vi "SaveDeviceHeader.vi"(0 "File Refnum in":refnum<file>, 1 "Comments":string, 5 "Filename":string, 7 "Run Number":i32, 9 "Array Titles":string, 11 "error in (no error)":errorcluster, 12 "Temperature":dbl, 13 "Humidity":dbl, 14 "Strip Segment":string) -> (4 "File Refnum out":refnum<file>, 6 "Header string":string, 10 "error out":errorcluster)   [LabVIEW 2013]
uses:
  globals/QC_RunInformation.vi
  globals/QC_MeasurementSetup.vi
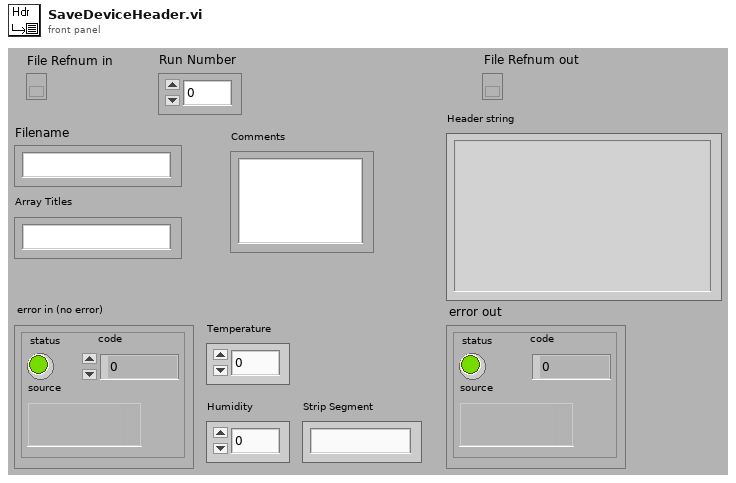
[diagram p1: front panel]
types:
  T1 = cluster{"Sensor Serial No.:":string, "Wafer:":string, "Batch:":string, "Manufacturer:":string, "Device Category:":string, "Database Serial No.:":string, "Date Initiated:":string, "Time Initiated:":string, "Test":string, "Probeplan used:":string, "End of Run comment:":string, "User:":string, "Vbias SMU":string, "LCR":string, "Test SMU":string, "Test DMM":string}
  T2 = cluster{"Institute":string, "Manufacturers":string[], "Devices":string[], "Serialnumbers Lookup DB":string, "Data directory":string, "Backup & screenshot directory":string, "List of known users":string[], "Measurement switch not used":bool, "Measurement Switch":string, "DUT Switch":string, "Rseries IV [MOhm]":string, "Rshunt IV [MOhm]":string, "Rseries CV [MOhm]":string, "DC blocking Cap [µF]":string, "Rseries LCR [MOhm]":string, "Rseries stability [MOhm]":string, "Rshunt stability [MOhm]":string, "Rseries striptest bias [MOhm]":string, "Rseries strip pinhole [MOhm]":string}
  T3 = cluster{"Supply":refnum<class "SupplyControl.lvclass">, "LCR":refnum<class "LCRControl.lvclass">, "Arduino":refnum<class "ArduinoControl.lvclass">, "Measurement switch":refnum<class "Switching.lvclass">, "Initial Voltage [V]":dbl, "Final Voltage [V]":dbl, "Step Size [V]":dbl, "Step Interval [s]":i32, "Number Of Steps":u32, "AC frequency [Hz]":i32, "RC Configuration":u16, "AC amplitude [V]":dbl, "Ramp down steps [V]":dbl, "Ramp down Interval [s]":i32, "Set Current Limit?":bool, "Current Limit [µA]":dbl, "Temperature Readout":enum16{"Read Arduino", "Enter manually"}, "Supply Name":string, "LCR Name":string, "V_depletion Limit [V]":dbl, "Measurement switch used?":bool}
  T4 = cluster{"Bias Supply":refnum<class "SupplyControl.lvclass">, "SMU":refnum<class "SupplyControl.lvclass">, "LCR":refnum<class "LCRControl.lvclass">, "ProbeStation":refnum<class "ProbeStationControl.lvclass">, "Arduino":refnum<class "ArduinoControl.lvclass">, "Measurement switch":refnum<class "Switching.lvclass">, "Probe Card Channels":i32, "Bias Voltage [V]":dbl, "First strip":i32, "Last strip":i32, "Base Voltage [V]":dbl, "Base Ramp Step [V]":dbl, "Base Ramp Interval [ms]":u32, "High Voltage [V]":dbl, "High Ramp Step [V]":dbl, "High Ramp Interval [ms]":u32, "AC frequency [Hz]":i32, "AC amplitude [V]":dbl, "RC Configuration":u16, "Single Needle":bool, "Temperature Readout":enum16{"Read Arduino", "Enter manually"}, "Fraction of good strips [%]":dbl, "Measurement switch used?":bool, "Matrix X Channels":cluster{"Mux1 C1":i32, "Mux1 C2":i32, "Mux2 C1":i32, "Mux2 C2":i32}, "Pinholes Y/N":bool, "Capacitance Y/N":bool, "Resistance Y/N":bool, "Bias Supply Name":string, "SMU Name":string, "LCR Name":string}
  T5 = cluster{"Supply":refnum<class "SupplyControl.lvclass">, "LCR":refnum<class "LCRControl.lvclass">, "Arduino":refnum<class "ArduinoControl.lvclass">, "Measurement switch":refnum<class "Switching.lvclass">, "Initial Voltage [V]":dbl, "Final Voltage [V]":dbl, "Step Size [V]":dbl, "Step Interval [s]":i32, "Number Of Steps":u32, "AC frequency [Hz]":i32, "RC Configuration":u16, "AC amplitude [V]":dbl, "Ramp down steps [V]":dbl, "Ramp down Interval [s]":i32, "Set Current Limit?":bool, "Current Limit [µA]":dbl, "Temperature Readout":enum16{"Read Arduino", "Enter manually"}, "Supply Name":string, "LCR Name":string, "C_is Limit [pF/cm]":dbl, "Measurement switch used?":bool}
  T6 = cluster{"Bias Supply":refnum<class "SupplyControl.lvclass">, "SMU":refnum<class "SupplyControl.lvclass">, "Arduino":refnum<class "ArduinoControl.lvclass">, "Initial Voltage [V]":dbl, "Final Voltage [V]":dbl, "Step Size [V]":dbl, "Step Interval [s]":i32, "Number Of Steps":u32, "Ramp down steps [V]":dbl, "Ramp down Interval [s]":i32, "Bias Voltage [V]":dbl, "Set Current Limit?":bool, "Current Limit [µA]":dbl, "Temperature Readout":enum16{"Read Arduino", "Enter manually"}, "Bias Supply Name":string, "SMU Name":string}
  T7 = cluster{"Supply":refnum<class "SupplyControl.lvclass">, "DMM":refnum<class "MultimeterControl.lvclass">, "DUT switch":refnum<class "Switching.lvclass">, "Arduino":refnum<class "ArduinoControl.lvclass">, "Measurement switch":refnum<class "Switching.lvclass">, "Voltage [V]":dbl, "Measurement Interval [s]":i32, "Test Duration":u32, "Ramp up steps [V]":dbl, "Ramp up Interval [s]":u32, "Ramp down steps [V]":dbl, "Ramp down Interval [s]":i32, "Set Current Limit?":bool, "Current Limit [µA]":dbl, "Temperature Readout":enum16{"Read Arduino", "Enter manually"}, "Supply Name":string, "DMM Name":string, "Maximum current fluctuation [%]":dbl, "Measurement switch used?":bool, "DUT switch used?":bool}
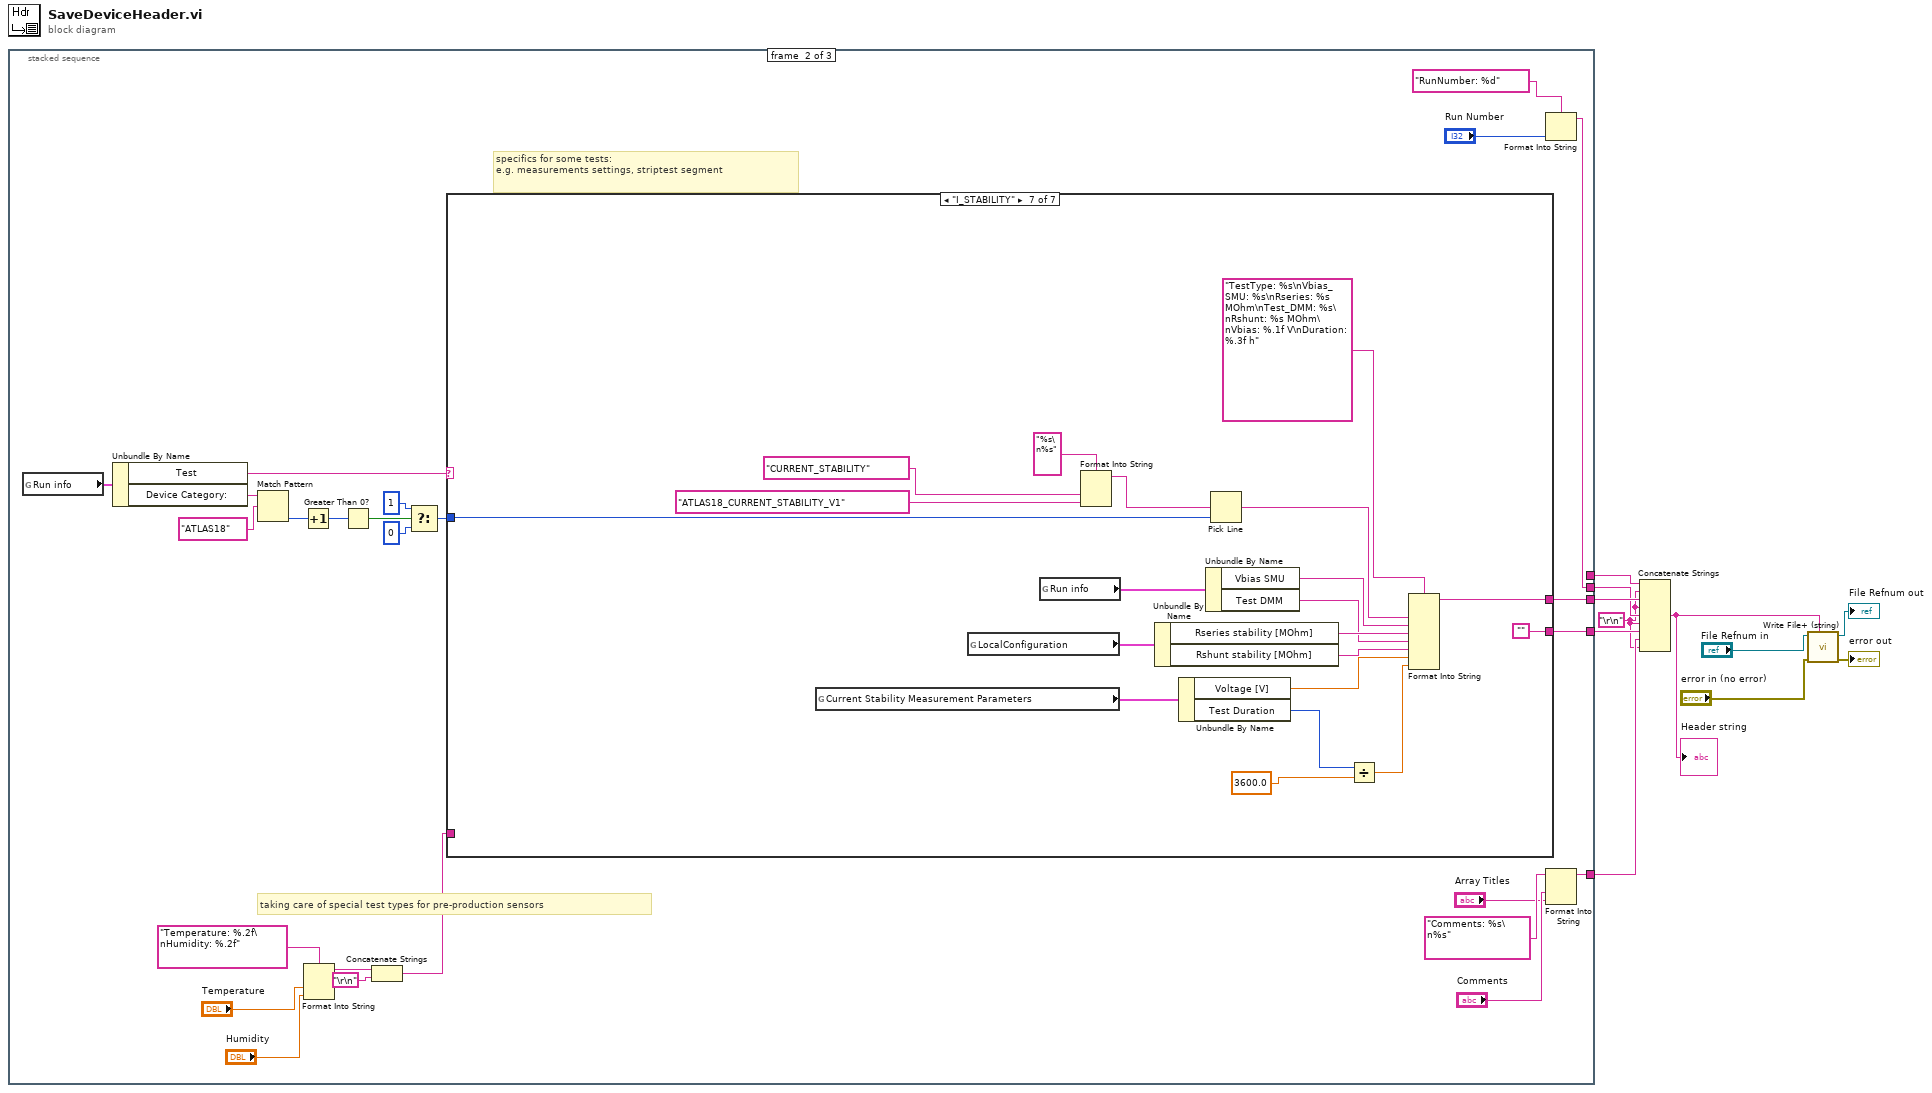
[diagram p0: block diagram]
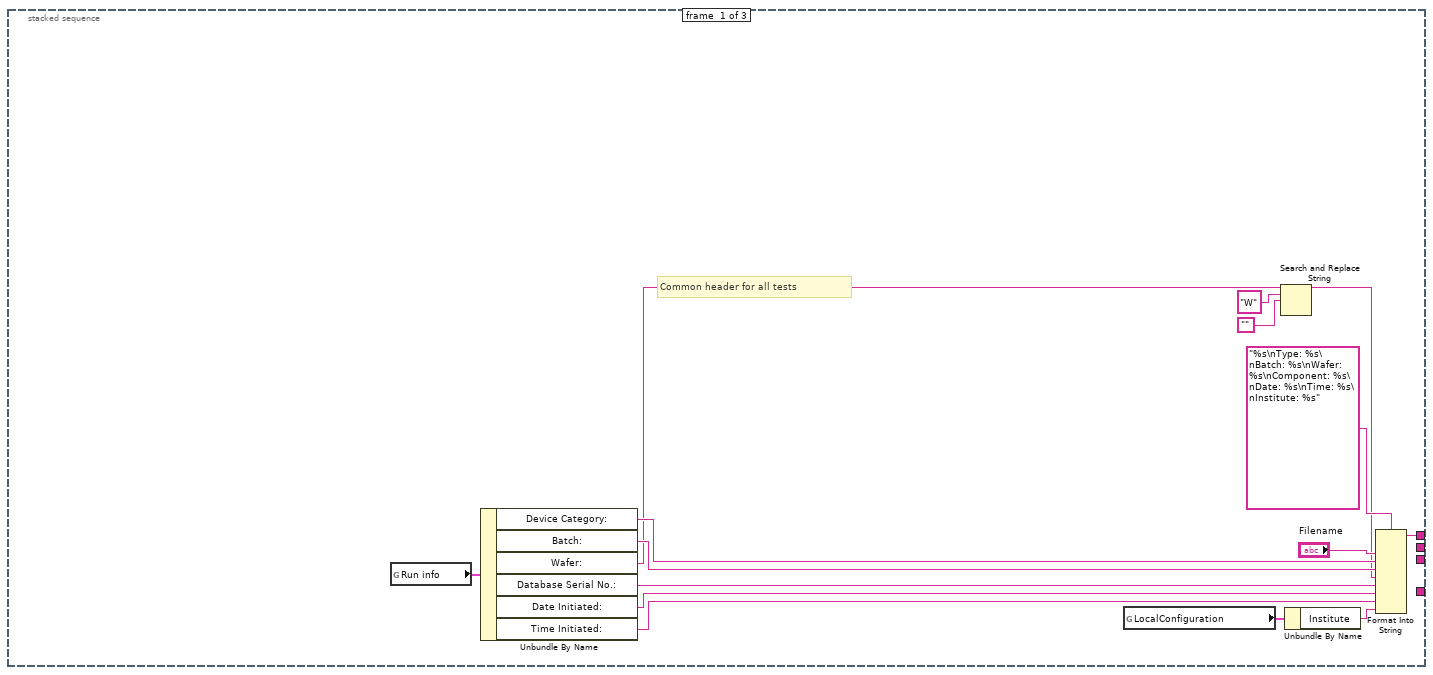
[diagram p2: hidden frame]
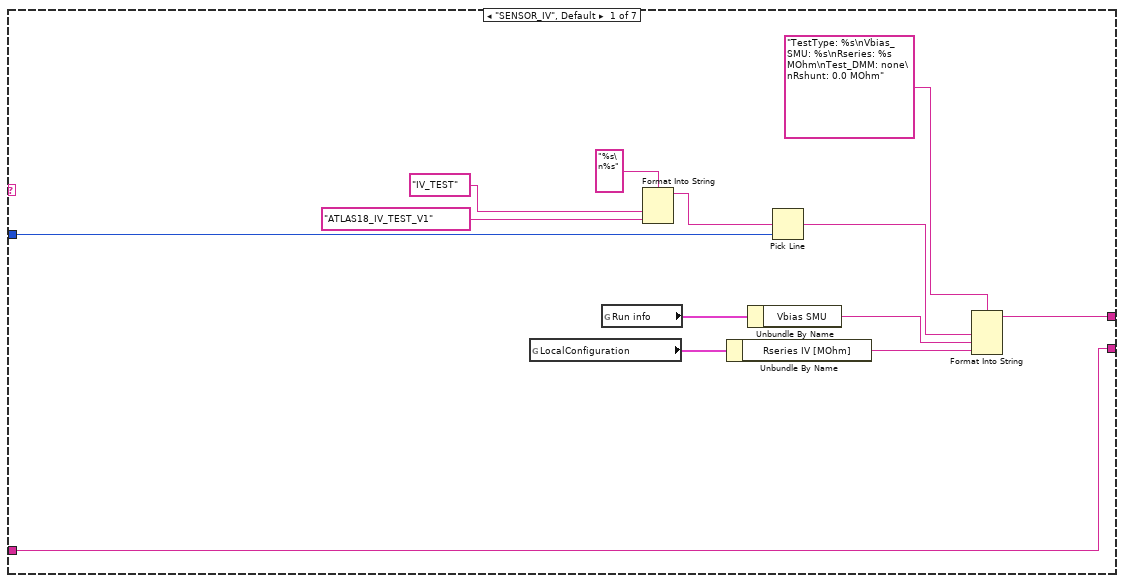
[diagram p3: hidden frame]
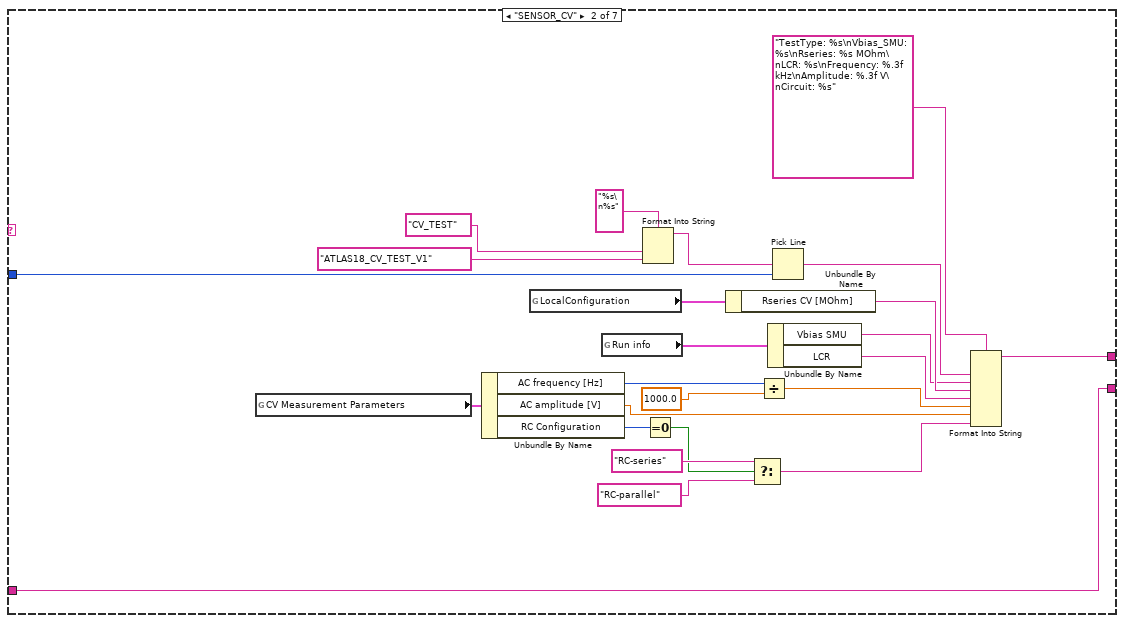
[diagram p4: hidden frame]
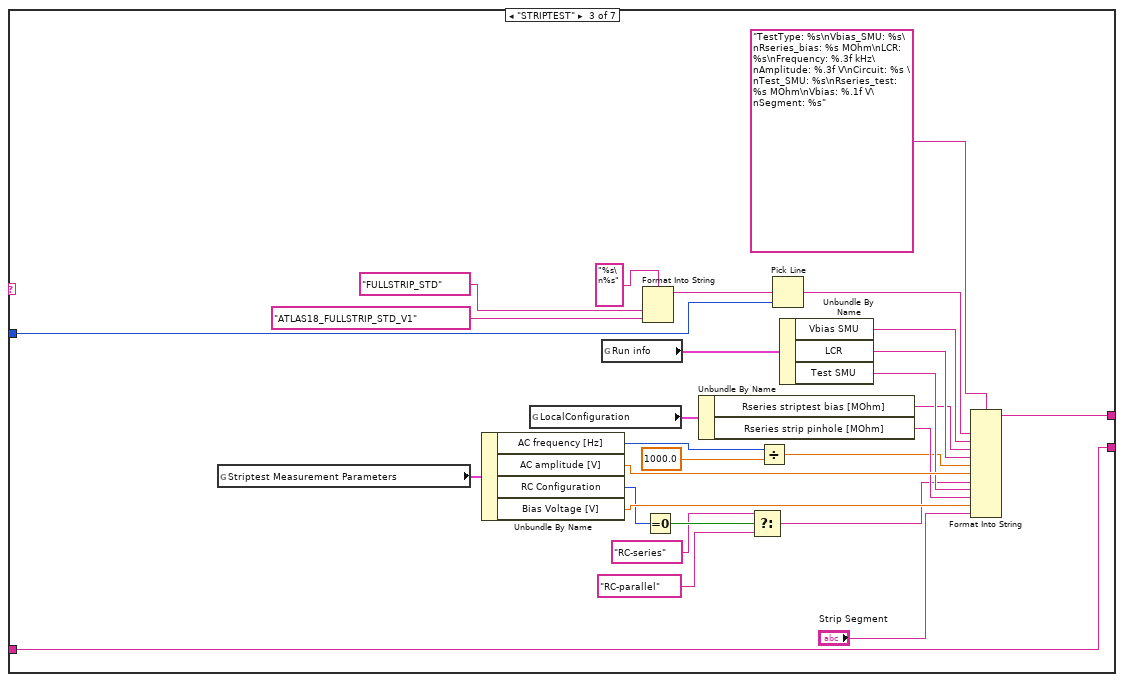
[diagram p5: hidden frame]
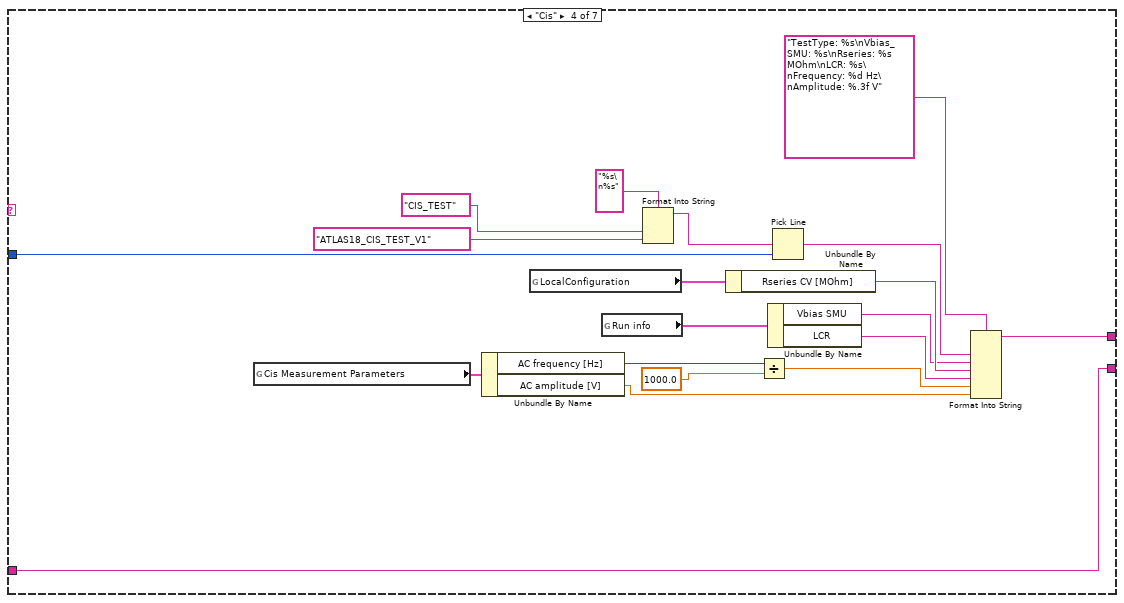
[diagram p6: hidden frame]
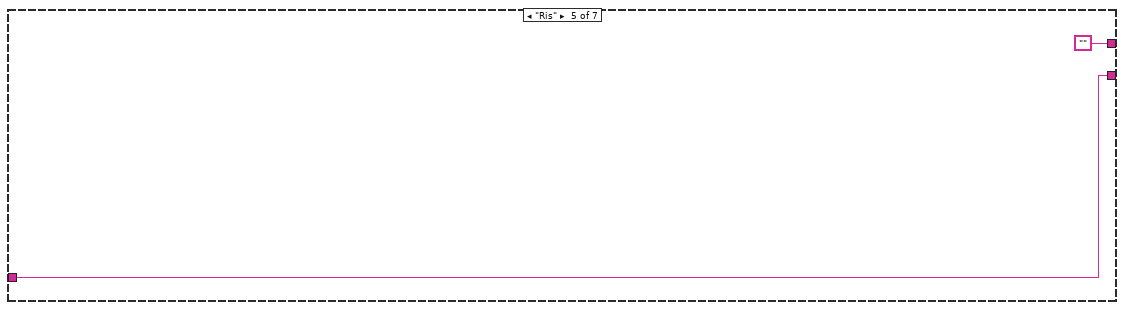
[diagram p7: hidden frame]
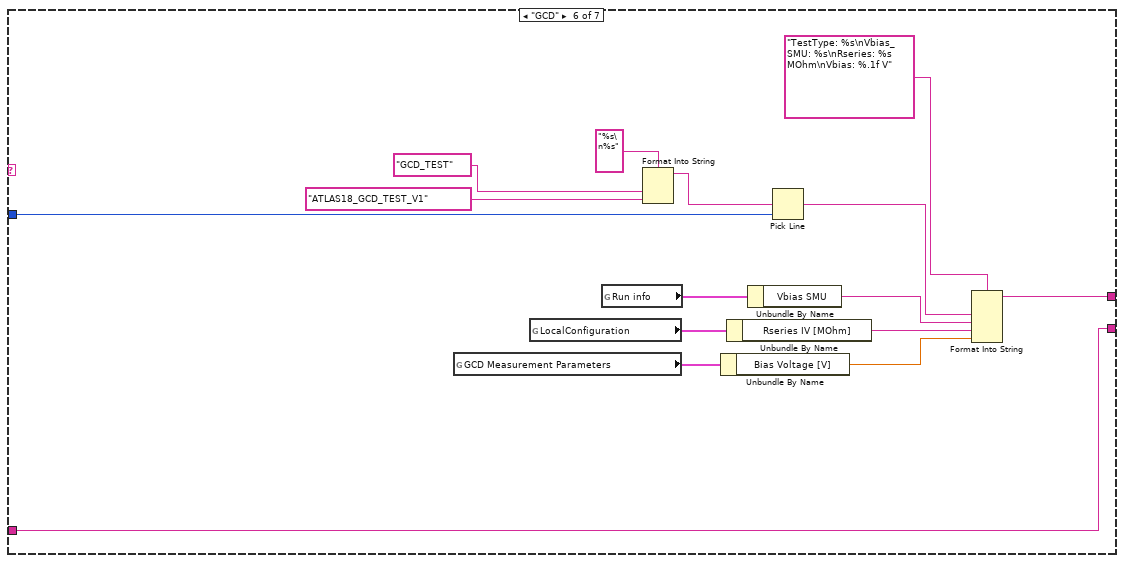
[diagram p8: hidden frame]
diagram:
  w1 = "\r\n"
  n1 = stacked-sequence {
    tunnel: [_ w51 _] -> w7
    tunnel: [_ w32 _] -> w6
    tunnel: [w16 _ _] -> w5
    tunnel: [_ w27 _] -> w3
    tunnel: [_ w31 _] -> w2
    frame #0 {
      # "Common header for all tests"
      n2 = global read "QC_RunInformation.vi" "Run info"() -> (w18:T1)
      n3 = Unbundle By Name(w18) -> ("Device Category:"=w21:string, "Batch:"=w22:string, "Wafer:"=w12:string, "Database Serial No.:"=w23:string, "Date Initiated:"=w24:string, "Time Initiated:"=w25:string)
      n4 = global read "QC_RunInformation.vi" "LocalConfiguration"() -> (w17:T2)
      n5 = Search and Replace String(input string=w12, search string="W", replace string="") -> (result string=w13:string)  [unwired: 5 in, 3 out]
      n6 = Unbundle By Name(w17) -> ("Institute"=w26:string)
      n7 = Format Into String(format string="%s\nType: %s\nBatch: %s\nWafer: %s\nComponent: %s\nDate: %s\nTime: %s\nInstitute: %s", "Filename", w21, w22, w13, w23, w24, w25, w26) -> (resulting string=w16:string)  [unwired: 2 in, 1 out]
    }
    frame #1 {
      # "taking care of special test types for pre-production sensors"
      # "specifics for some tests:\ne.g. measurements settings, striptest segment"
      n8 = global read "QC_RunInformation.vi" "Run info"() -> (w50:T1)
      n9 = Unbundle By Name(w50) -> ("Test"=w49:string, "Device Category:"=w44:string)
      n10 = Match Pattern(string=w44, regular expression="ATLAS18") -> (offset past match=w46:i32)  [unwired: 1 in, 3 out]
      n11 = Increment(x=w46) -> (x+1=w47:i32)
      n12 = Format Into String(format string="Temperature: %.2f\nHumidity: %.2f", "Temperature", "Humidity") -> (resulting string=w29:string)  [unwired: 2 in, 1 out]
      n13 = Greater Than 0?(x=w47) -> (x > 0?=w48:bool)
      n14 = Concatenate Strings(w29, "\r\n") -> (w28:string)
      n15 = Select(t=1, s=w48, f=0) -> (s? t:f=w41:i32)
      n16 = case shown="\"I_STABILITY\"" w49 {
        tunnel: [w60 w81 w113 w128 "" w146 w168] -> w51
        tunnel: w41 -> [w56 w76 w94 w123 _ w141 w159]
        tunnel: w28 -> [w52 w65 w89 w117 w136 w138 _]
        tunnel: [w52 w65 w89 w117 w136 w138 ""] -> w27
        frame "SENSOR_IV", Default {
          n17 = global read "QC_RunInformation.vi" "LocalConfiguration"() -> (w64:T2)
          n18 = global read "QC_RunInformation.vi" "Run info"() -> (w63:T1)
          n19 = Format Into String(format string="%s\n%s", "IV_TEST", "ATLAS18_IV_TEST_V1") -> (resulting string=w57:string)  [unwired: 2 in, 1 out]
          n20 = Unbundle By Name(w64) -> ("Rseries IV [MOhm]"=w61:string)
          n21 = Unbundle By Name(w63) -> ("Vbias SMU"=w59:string)
          n22 = Pick Line(multi-line string=w57, line index=w56) -> (output string=w53:string)  [unwired: 1 in]
          n23 = Format Into String(format string="TestType: %s\nVbias_SMU: %s\nRseries: %s MOhm\nTest_DMM: none\nRshunt: 0.0 MOhm", w53, w59, w61) -> (resulting string=w60:string)  [unwired: 2 in, 1 out]
        }
        frame "SENSOR_CV" {
          n24 = global read "QC_MeasurementSetup.vi" "CV Measurement Parameters"() -> (w88:T3)
          n25 = Unbundle By Name(w88) -> ("AC frequency [Hz]"=w67:i32, "AC amplitude [V]"=w82:dbl, "RC Configuration"=w73:u16)
          n26 = global read "QC_RunInformation.vi" "LocalConfiguration"() -> (w87:T2)
          n27 = global read "QC_RunInformation.vi" "Run info"() -> (w86:T1)
          n28 = Format Into String(format string="%s\n%s", "CV_TEST", "ATLAS18_CV_TEST_V1") -> (resulting string=w77:string)  [unwired: 2 in, 1 out]
          n29 = Equal To 0?(x=w73) -> (x = 0?=w70:bool)
          n30 = Unbundle By Name(w87) -> ("Rseries CV [MOhm]"=w84:string)
          n31 = Select(t="RC-series", s=w70, f="RC-parallel") -> (s? t:f=w69:string)
          n32 = Divide(x=w67, y=1000.0) -> (x/y=w66:dbl)
          n33 = Unbundle By Name(w86) -> ("Vbias SMU"=w75:string, "LCR"=w83:string)
          n34 = Pick Line(multi-line string=w77, line index=w76) -> (output string=w74:string)  [unwired: 1 in]
          n35 = Format Into String(format string="TestType: %s\nVbias_SMU: %s\nRseries: %s MOhm\nLCR: %s\nFrequency: %.3f kHz\nAmplitude: %.3f V\nCircuit: %s", w74, w75, w84, w83, w66, w82, w69) -> (resulting string=w81:string)  [unwired: 2 in, 1 out]
        }
        frame "STRIPTEST" {
          n36 = global read "QC_MeasurementSetup.vi" "Striptest Measurement Parameters"() -> (w115:T4)
          n37 = Unbundle By Name(w115) -> ("AC frequency [Hz]"=w91:i32, "AC amplitude [V]"=w112:dbl, "RC Configuration"=w104:u16, "Bias Voltage [V]"=w106:dbl)
          n38 = global read "QC_RunInformation.vi" "LocalConfiguration"() -> (w108:T2)
          n39 = global read "QC_RunInformation.vi" "Run info"() -> (w116:T1)
          n40 = Format Into String(format string="%s\n%s", "FULLSTRIP_STD", "ATLAS18_FULLSTRIP_STD_V1") -> (resulting string=w95:string)  [unwired: 2 in, 1 out]
          n41 = Equal To 0?(x=w104) -> (x = 0?=w103:bool)
          n42 = Unbundle By Name(w108) -> ("Rseries striptest bias [MOhm]"=w107:string, "Rseries strip pinhole [MOhm]"=w105:string)
          n43 = Select(t="RC-series", s=w103, f="RC-parallel") -> (s? t:f=w100:string)
          n44 = Divide(x=w91, y=1000.0) -> (x/y=w90:dbl)
          n45 = Pick Line(multi-line string=w95, line index=w94) -> (output string=w93:string)  [unwired: 1 in]
          n46 = Unbundle By Name(w116) -> ("Vbias SMU"=w99:string, "LCR"=w110:string, "Test SMU"=w109:string)
          n47 = Format Into String(format string="TestType: %s\nVbias_SMU: %s\nRseries_bias: %s MOhm\nLCR: %s\nFrequency: %.3f kHz\nAmplitude: %.3f V\nCircuit: %s \nTest_SMU: %s\nRseries_test: %s MOhm\nVbias: %.1f V\nSegment: %s", w93, w99, w107, w110, w90, w112, w100, w109, w105, w106, "Strip Segment") -> (resulting string=w113:string)  [unwired: 2 in, 1 out]
        }
        frame "Cis" {
          n48 = global read "QC_MeasurementSetup.vi" "Cis Measurement Parameters"() -> (w135:T5)
          n49 = Unbundle By Name(w135) -> ("AC frequency [Hz]"=w119:i32, "AC amplitude [V]"=w129:dbl)
          n50 = global read "QC_RunInformation.vi" "LocalConfiguration"() -> (w134:T2)
          n51 = global read "QC_RunInformation.vi" "Run info"() -> (w133:T1)
          n52 = Format Into String(format string="%s\n%s", "CIS_TEST", "ATLAS18_CIS_TEST_V1") -> (resulting string=w124:string)  [unwired: 2 in, 1 out]
          n53 = Unbundle By Name(w134) -> ("Rseries CV [MOhm]"=w131:string)
          n54 = Divide(x=w119, y=1000.0) -> (x/y=w118:dbl)
          n55 = Unbundle By Name(w133) -> ("Vbias SMU"=w122:string, "LCR"=w130:string)
          n56 = Pick Line(multi-line string=w124, line index=w123) -> (output string=w121:string)  [unwired: 1 in]
          n57 = Format Into String(format string="TestType: %s\nVbias_SMU: %s\nRseries: %s MOhm\nLCR: %s\nFrequency: %d Hz\nAmplitude: %.3f V", w121, w122, w131, w130, w118, w129) -> (resulting string=w128:string)  [unwired: 2 in, 1 out]
        }
        frame "Ris" {
        }
        frame "GCD" {
          n58 = global read "QC_MeasurementSetup.vi" "GCD Measurement Parameters"() -> (w148:T6)
          n59 = global read "QC_RunInformation.vi" "LocalConfiguration"() -> (w152:T2)
          n60 = global read "QC_RunInformation.vi" "Run info"() -> (w151:T1)
          n61 = Format Into String(format string="%s\n%s", "GCD_TEST", "ATLAS18_GCD_TEST_V1") -> (resulting string=w142:string)  [unwired: 2 in, 1 out]
          n62 = Unbundle By Name(w148) -> ("Bias Voltage [V]"=w147:dbl)
          n63 = Unbundle By Name(w152) -> ("Rseries IV [MOhm]"=w149:string)
          n64 = Unbundle By Name(w151) -> ("Vbias SMU"=w140:string)
          n65 = Pick Line(multi-line string=w142, line index=w141) -> (output string=w139:string)  [unwired: 1 in]
          n66 = Format Into String(format string="TestType: %s\nVbias_SMU: %s\nRseries: %s MOhm\nVbias: %.1f V", w139, w140, w149, w147) -> (resulting string=w146:string)  [unwired: 2 in, 1 out]
        }
        frame "I_STABILITY" {
          n67 = global read "QC_MeasurementSetup.vi" "Current Stability Measurement Parameters"() -> (w172:T7)
          n68 = global read "QC_RunInformation.vi" "LocalConfiguration"() -> (w171:T2)
          n69 = global read "QC_RunInformation.vi" "Run info"() -> (w170:T1)
          n70 = Format Into String(format string="%s\n%s", "CURRENT_STABILITY", "ATLAS18_CURRENT_STABILITY_V1") -> (resulting string=w160:string)  [unwired: 2 in, 1 out]
          n71 = Unbundle By Name(w171) -> ("Rseries stability [MOhm]"=w167:string, "Rshunt stability [MOhm]"=w165:string)
          n72 = Unbundle By Name(w172) -> ("Voltage [V]"=w164:dbl, "Test Duration"=w154:u32)
          n73 = Unbundle By Name(w170) -> ("Vbias SMU"=w158:string, "Test DMM"=w166:string)
          n74 = Pick Line(multi-line string=w160, line index=w159) -> (output string=w157:string)  [unwired: 1 in]
          n75 = Divide(x=w154, y=3600.0) -> (x/y=w153:dbl)
          n76 = Format Into String(format string="TestType: %s\nVbias_SMU: %s\nRseries: %s MOhm\nTest_DMM: %s\nRshunt: %s MOhm\nVbias: %.1f V\nDuration: %.3f h", w157, w158, w167, w166, w165, w164, w153) -> (resulting string=w168:string)  [unwired: 2 in, 1 out]
        }
      }
      n77 = Format Into String(format string="RunNumber: %d", "Run Number") -> (resulting string=w32:string)  [unwired: 2 in, 1 out]
      n78 = Format Into String(initial string="Comments: %s\n%s", "Comments", "Array Titles") -> (resulting string=w31:string)  [unwired: 2 in, 1 out]
    }
    frame #2 {
    }
  }
  n79 = Concatenate Strings(w5, w1, w7, w1, w6, w1, w3, w2, w1) -> (w4:string)
  "Header string" <- w4
  n80 = call <vilib>:"Write File+ (string).vi"("string"=w4, "error in (no error)"="error in (no error)", "refnum"="File Refnum in") -> ("error out"=→"error out":errorcluster, "dup refnum"=→"File Refnum out":refnum<file>)  [unwired: 4 in, 1 out]
